vi "WriteVIDictionary.vi"(7 "Additional Languages":string[](array[string]), 8 "error in (no error)":errorcluster, 9 "Current VI Language":string, 10 "Dictionary Path":path, 11 "VI in":refnum<vi>) -> (0 "error out":errorcluster, 3 "Text to Write (for debug)":string)   [LabVIEW 2017]
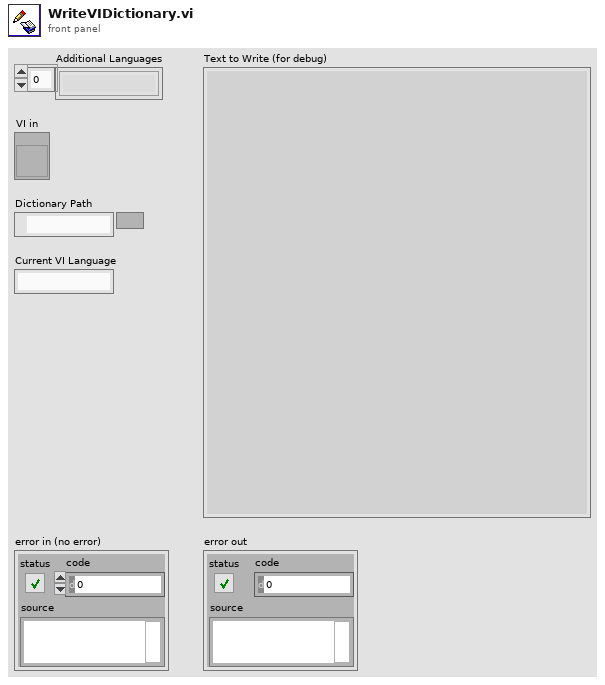
[diagram p1: front panel]
types:
  T1 = enum16{"open", "replace", "create", "open or create", "replace or create", "replace or create with confirmation"}
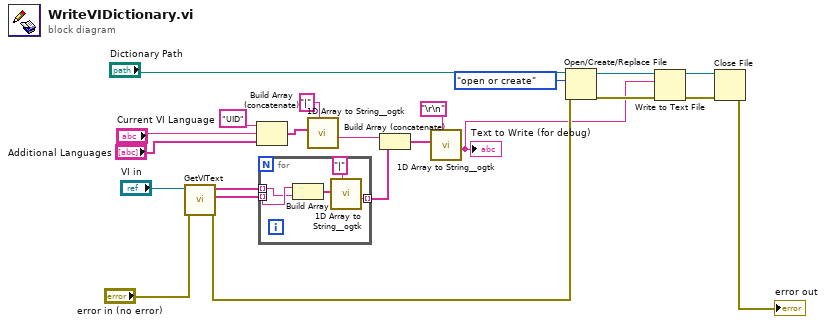
[diagram p0: block diagram]
diagram:
  n1 = call "GetVIText.vi"("error in (no error)"="error in (no error)", "VI"="VI in") -> ("error out"=w18:errorcluster, "Control UIDs"=w6:string[], "Control Text"=w5:string[])  [unwired: 7 in]
  n2 = Build Array (concatenate)("UID" ("element"), "Current VI Language", "Additional Languages") -> (w7:string[])
  n3 = for {
    tunnel: w5 -> [w23] mode=indexing
    tunnel: w6 -> [w24] mode=indexing
    tunnel: [w25] -> w11 mode=indexing
    n4 = Build Array(w24, w23) -> (w27:string[])
    n5 = call <userlib>:"1D Array to String__ogtk.vi"("delimiter (Tab)"="|", "Array of Strings"=w27) -> ("delimited string"=w25:string)  [unwired: 9 in]
  }
  n6 = call <userlib>:"1D Array to String__ogtk.vi"("delimiter (Tab)"="|", "Array of Strings"=w7) -> ("delimited string"=w10:string)  [unwired: 9 in]
  n7 = Build Array (concatenate)(w10, w11) -> (w12:string[])
  n8 = call <userlib>:"1D Array to String__ogtk.vi"("delimiter (Tab)"="\r\n", "Array of Strings"=w12) -> ("delimited string"=w16:string)  [unwired: 9 in]
  "Text to Write (for debug)" <- w16
  n9 = Open/Create/Replace File(file path (use dialog)="Dictionary Path", error in=w18, operation (0:open)=T1."open or create") -> (refnum out=w15:refnum<file>, error out=w19:errorcluster)  [unwired: 3 in, 1 out]
  n10 = Write to Text File(file (use dialog)=w15, text=w16, error in=w19) -> (refnum out=w21:refnum<file>, error out=w20:errorcluster)  [unwired: 1 in, 1 out]
  n11 = Close File(refnum=w21, error in=w20) -> (error out=→"error out":errorcluster)  [unwired: 1 out]
